vi "Do.vi"(8 "error in":errorcluster, 10 "Actor in":refnum<class "Actor.lvclass">, 11 "Update Housekeeping MSG":refnum<class "Update Housekeeping MSG.lvclass">) -> (0 "error out":errorcluster, 2 "Actor out":refnum<class "Actor.lvclass">)   [LabVIEW 2018, in "eCRDS Library.lvlib" / "Update Housekeeping MSG.lvclass"]
doc: "(<B>Filename</B>: Actor Framework.lvlib:Message.lvclass:Do.vi)\n\nDefines what a message does when it is received by an actor. Generally, a message instructs an actor to invoke one of its methods. By default, this method does nothing. A child class must override it to define behavior. Create a child class by using the Actor Framework Message Maker dialog box."
uses:
  Update Housekeeping MSG.lvclass
  <vilib>/ActorFramework/Actor/Actor.lvclass
  Update Housekeeping MSG.lvclass/Update Housekeeping MSG.ctl
  CRDS/Main/eCRDS.lvclass
  C:/Users/Labview/Documents/exscalabar_server/reusable/Instrument/Instrument.lvclass
  Instr Actor.lvclass
  C:/Program Files (x86)/National Instruments/LabVIEW 2018/vi.lib/ActorFramework/Actor/Actor.lvclass
  Instr Actor.lvclass/Instr Actor.ctl
  CRDS/Main/eCRDS.lvclass/eCRDS.ctl
  reusable/Instrument/Instrument.lvclass/Instrument.ctl
  Accessors/Read Instr.vi
  CRDS/Main/Accessors/Read HK DVR.vi
  reusable/Instrument/Read Log Session.vi
  reusable/Instrument/Instrument.lvclass
  <userlib>/_Session Fwk/Session - Root.lvclass
  reusable/Session APIs/Session Log/System Log.lvclass
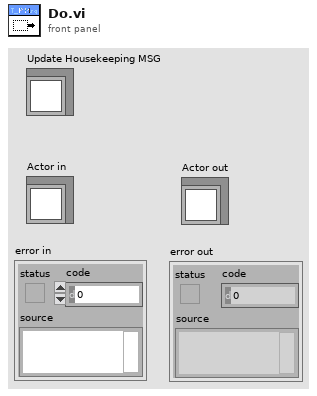
[diagram p1: front panel]
types:
  T1 = cluster{"T (degC)":dbl, "P (mb)":dbl, "Q (lpm)":dbl}[]
  T2 = typedef "Session - Root.lvclass/Session Handle.ctl" = refnum<data-value>
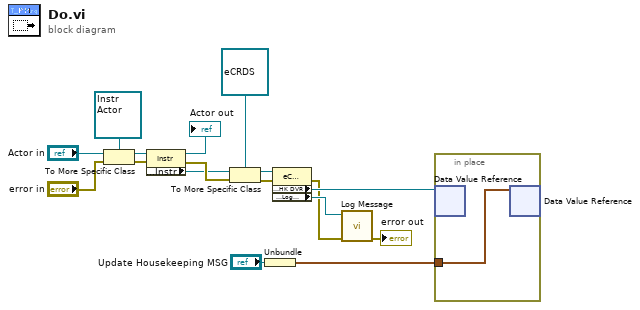
[diagram p0: block diagram]
diagram:
  n1 = To More Specific Class(target class=refnum<class "Instr Actor.lvclass"> refnum ("Instrument Lib:Instr"), reference="Actor in", error in="error in") -> (specific class reference=w15:refnum<class "Instr Actor.lvclass">, error out=w5:errorcluster)
  n2 = property class="Instr"(reference=w15, error in=w5) -> (reference out=→"Actor out":refnum<class "Instr Actor.lvclass">, error out=w14:errorcluster, "Accessors:Instr"=w13:refnum<class "Instrument.lvclass">)
  n3 = To More Specific Class(target class=refnum<class "eCRDS.lvclass"> refnum ("eCRDS"), reference=w13, error in=w14) -> (specific class reference=w11:refnum<class "eCRDS.lvclass">, error out=w7:errorcluster)
  n4 = Unbundle("Update Housekeeping MSG") -> (w8:T1)
  n5 = property class="eCRDS"(reference=w11, error in=w7) -> (error out=w1:errorcluster, "Accessors:HK DVR"=w10:refnum<data-value>, "Accessors:Log Session"=w3:T2)  [unwired: 1 out]
  n6 = call "Log Message.vi"("error in"=w1, "session in"=w3) -> ("error out"=→"error out":errorcluster)  [unwired: 8 in, 1 out]
  n7 = in-place {
    in-place-border: w8 -> [w18]
    n8 = in-place-dvr #1(w10) -> ()  [unwired: 2 out]
    n9 = in-place-dvr #1(w18) -> ()  [unwired: 2 out]
  }
